vi "Teleop.vi"(10 "Match Info":T1={"Autonomous Elapsed Seconds"=0.0, "TeleOp Elapsed Seconds"=0.0, "Disabled Elapsed Seconds"=0.0, "Visited Autonomous"=FALSE, "Visited TeleOp"=FALSE, "Visited Disabled"=FALSE, "Autonomous Settings"={"Autonomous Style"=enum."Independent", "VI Refnum"=refnum}}, 11 "Call Context":T2) -> ()   [LabVIEW 2015]
doc: "This VI is called for each TeleOp packet received from the DS where the robot is not disabled. It is often used to read from the joysticks and update I/O or to update setpoints for timed control loops. It should complete and return within 20 milliseconds or it may miss DS packets."
uses:
  <vilib>/Rock Robotics/WPI/DriverStation/WPI_DriverStationDerivedRobotMode.ctl
  <vilib>/Rock Robotics/WPI/DriverStation/WPI_DriverStationMatch Info.ctl
  <vilib>/Rock Robotics/WPI/Solenoid/WPI_SolenoidValue.ctl
  <vilib>/Rock Robotics/WPI/CAN/TalonSRX/WPI_CANTalonSRX_APIControlMode.ctl
  <vilib>/Rock Robotics/WPI/Utilities/WPI_GetSetVariantRefNum.vi
  Robot Global Data.vi
  <vilib>/Rock Robotics/WPI/Solenoid/WPI_SolenoidSetEnum.vi
  <vilib>/Rock Robotics/Network Tables/NT Write Boolean.vi
  <vilib>/addons/control/pid/pid.llb/PID (DBL).vi
  <vilib>/addons/control/pid/NI_PID_pid.lvlib
panel:
  out "Shooter velocity":dbl
  out "Shooter Applied Throttle":dbl
  out "Shooter Current":dbl
  out "Arm Pot":dbl
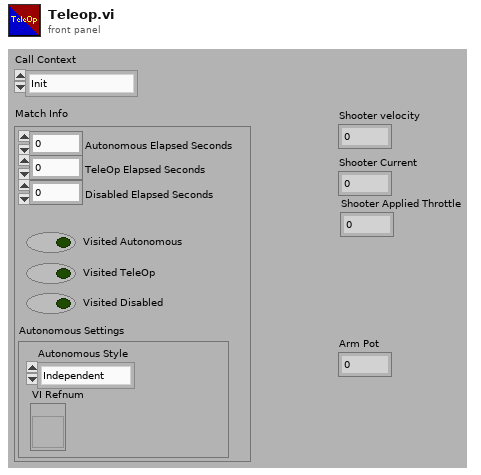
[diagram p1: front panel]
types:
  T1 = typedef "WPI_DriverStationMatch Info.ctl" = cluster{"Autonomous Elapsed Seconds":dbl, "TeleOp Elapsed Seconds":dbl, "Disabled Elapsed Seconds":dbl, "Visited Autonomous":bool, "Visited TeleOp":bool, "Visited Disabled":bool, "Autonomous Settings":cluster{"Autonomous Style":enum16{"Iterative", "Independent"}, "VI Refnum":refnum<vi>}}
  T2 = typedef "WPI_DriverStationDerivedRobotMode.ctl" = enum16{"Init", "Execute", "Stop"}
  T3 = typedef "WPI_SolenoidValue.ctl" = enum16{"Off", "On", "Forward", "Reverse"}
  T4 = typedef "WPI_JoystickDevRef.ctl" = cluster{"Device":T5}
  T5 = typedef "WPI_JoystickDeviceEnum.ctl" = enum16{"USB 0", "USB 1", "USB 2", "USB 3", "USB 4", "USB 5"}
  T6 = cluster{"Axes[0]":dbl, "Axes[1]":dbl, "Axes[2]":dbl, "Axes[3]":dbl, "Axes[4]":dbl, "Axes[5]":dbl, "Axes[6]":dbl, "Axes[7]":dbl, "Axes[8]":dbl}
  T7 = typedef "WPI_MotorControlDeviceRef.ctl" = cluster{"DeviceStatus":errorcluster, "Type":T8, "PWM":cluster{"PWM Channel":T9, "DeadBand":T10}, "CAN":cluster{"Device Number":u8, "Control Mode":T11, "Semaphore":T12, "Max Vout":dbl, "TalonSRX Control Mode":T13}, "Invert":bool}
  T8 = typedef "WPI_MotorControlType.ctl" = enum16{"PWM", "CAN", "CANTalonSRX"}
  T9 = typedef "FPGA_DIOPWMChannel.ctl" = enum8{"PWM 0", "PWM 1", "PWM 2", "PWM 3", "PWM 4", "PWM 5", "PWM 6", "PWM 7", "PWM 8", "PWM 9", "PWM MXP 0", "PWM MXP 1", "PWM MXP 2", "PWM MXP 3", "PWM MXP 4", "PWM MXP 5", "PWM MXP 6", "PWM MXP 7", "PWM MXP 8", "PWM MXP 9", "Invalid"}
  T10 = typedef "WPI_PWMDeadband.ctl" = cluster{"Name":string, "maxPositivePwm":i32, "minPositivePwm":i32, "centerPwm":i32, "maxNegativePwm":i32, "minNegativePwm":i32, "angularRange":u16}
  T11 = typedef "WPI_CANJaguar_ControlMode.ctl" = enum8{"Percent VBus", "Current", "Speed", "Position", "Voltage"}
  T12 = typedef "Semaphore RefNum" = refnum<k1>
  T13 = typedef "WPI_CANTalonSRX_APIControlMode.ctl" = enum8{"Percent VBus", "Speed", "Position", "Slave", "Unchanged / Invalid", "Voltage Compensation", "Current", "Motion Profile"}
  T14 = cluster{"Buttons[0]":bool, "Buttons[1]":bool, "Buttons[2]":bool, "Buttons[3]":bool, "Buttons[4]":bool, "Buttons[5]":bool, "Buttons[6]":bool, "Buttons[7]":bool, "Buttons[8]":bool}
  T15 = typedef "WPI_CompressorDevRef.ctl" = cluster{"DevStatus":errorcluster, "Pneumatics Control Module":u8}
  T16 = typedef "WPI_SolenoidDevRef.ctl" = cluster{"DevStatus":errorcluster, "Pneumatics Control Module":u8, "Forward Solenoid Channel":T17, "Reverse Solenoid Channel":T17}
  T17 = typedef "WPI_SolenoidChannel.ctl" = enum8{"Solenoid 0", "Solenoid 1", "Solenoid 2", "Solenoid 3", "Solenoid 4", "Solenoid 5", "Solenoid 6", "Solenoid 7", "Invalid"}
  T18 = typedef "WPI_CANTalonSRX_GlobalStatus.ctl" = cluster{"Applied Throttle":dbl, "Module Enabled":bool, "CAN Error":errorcluster, "Closed Loop Error":dbl, "Forward Limit Switch Closed":bool, "Reverse Limit Switch Closed":bool, "Sensor Position":dbl, "Sensor Velocity":dbl, "Current":dbl, "Sticky Fault - Over Temp":bool, "Sticky Fault - Under Voltage":bool, "Sticky Fault - Forward Limit":bool, "Sticky Fault - Reverse Limit":bool, "Sticky Fault - Forward Soft Limit":bool, "Sticky Fault - Reverse Soft Limit":bool, "Brake is Enabled":bool, "Encoder Position":dbl, "Encoder Velocity":dbl, "Encoder Index Count":dbl, "Encoder A Pin State":bool, "Encoder B Pin State":bool, "Encoder Index Pin State":bool, "Analog In":dbl, "Analog In Velocity":dbl, "Temperature (C)":dbl, "Battery Voltage":dbl, "Control 5 Is Supported":bool, "Current Profile Slot Select":dbl, "Pos Div 8":bool, "Vel Div 4":bool, "Pulse Width Position":i32, "Pulse Width Velocity":i32, "Pulse Width Rise To Rise (us)":i32, "Pulse Width Rise To Fall (us)":i32, "Mot Prof Active Is Under Run":bool, "Mot Prof Active Has Under Run":bool, "Mot Prof Active Is Last":bool, "Mot Prof Active Velocity Only":bool, "Mot Prof Active Is Valid":bool, "Mot Prof Buffer Is Full":bool, "Mot Prof Active Profile Slot Select":i32, "Mot Prof NextID":i32, "Mot Prof Count":i32, "Mot Prof Active Velocity":dbl, "Mot Prof Active Position":dbl, "Mot Prof Output Enable":i32}
  T19 = cluster{"proportional gain (Kc)":dbl, "integral time (Ti, min)":dbl, "derivative time (Td, min)":dbl}
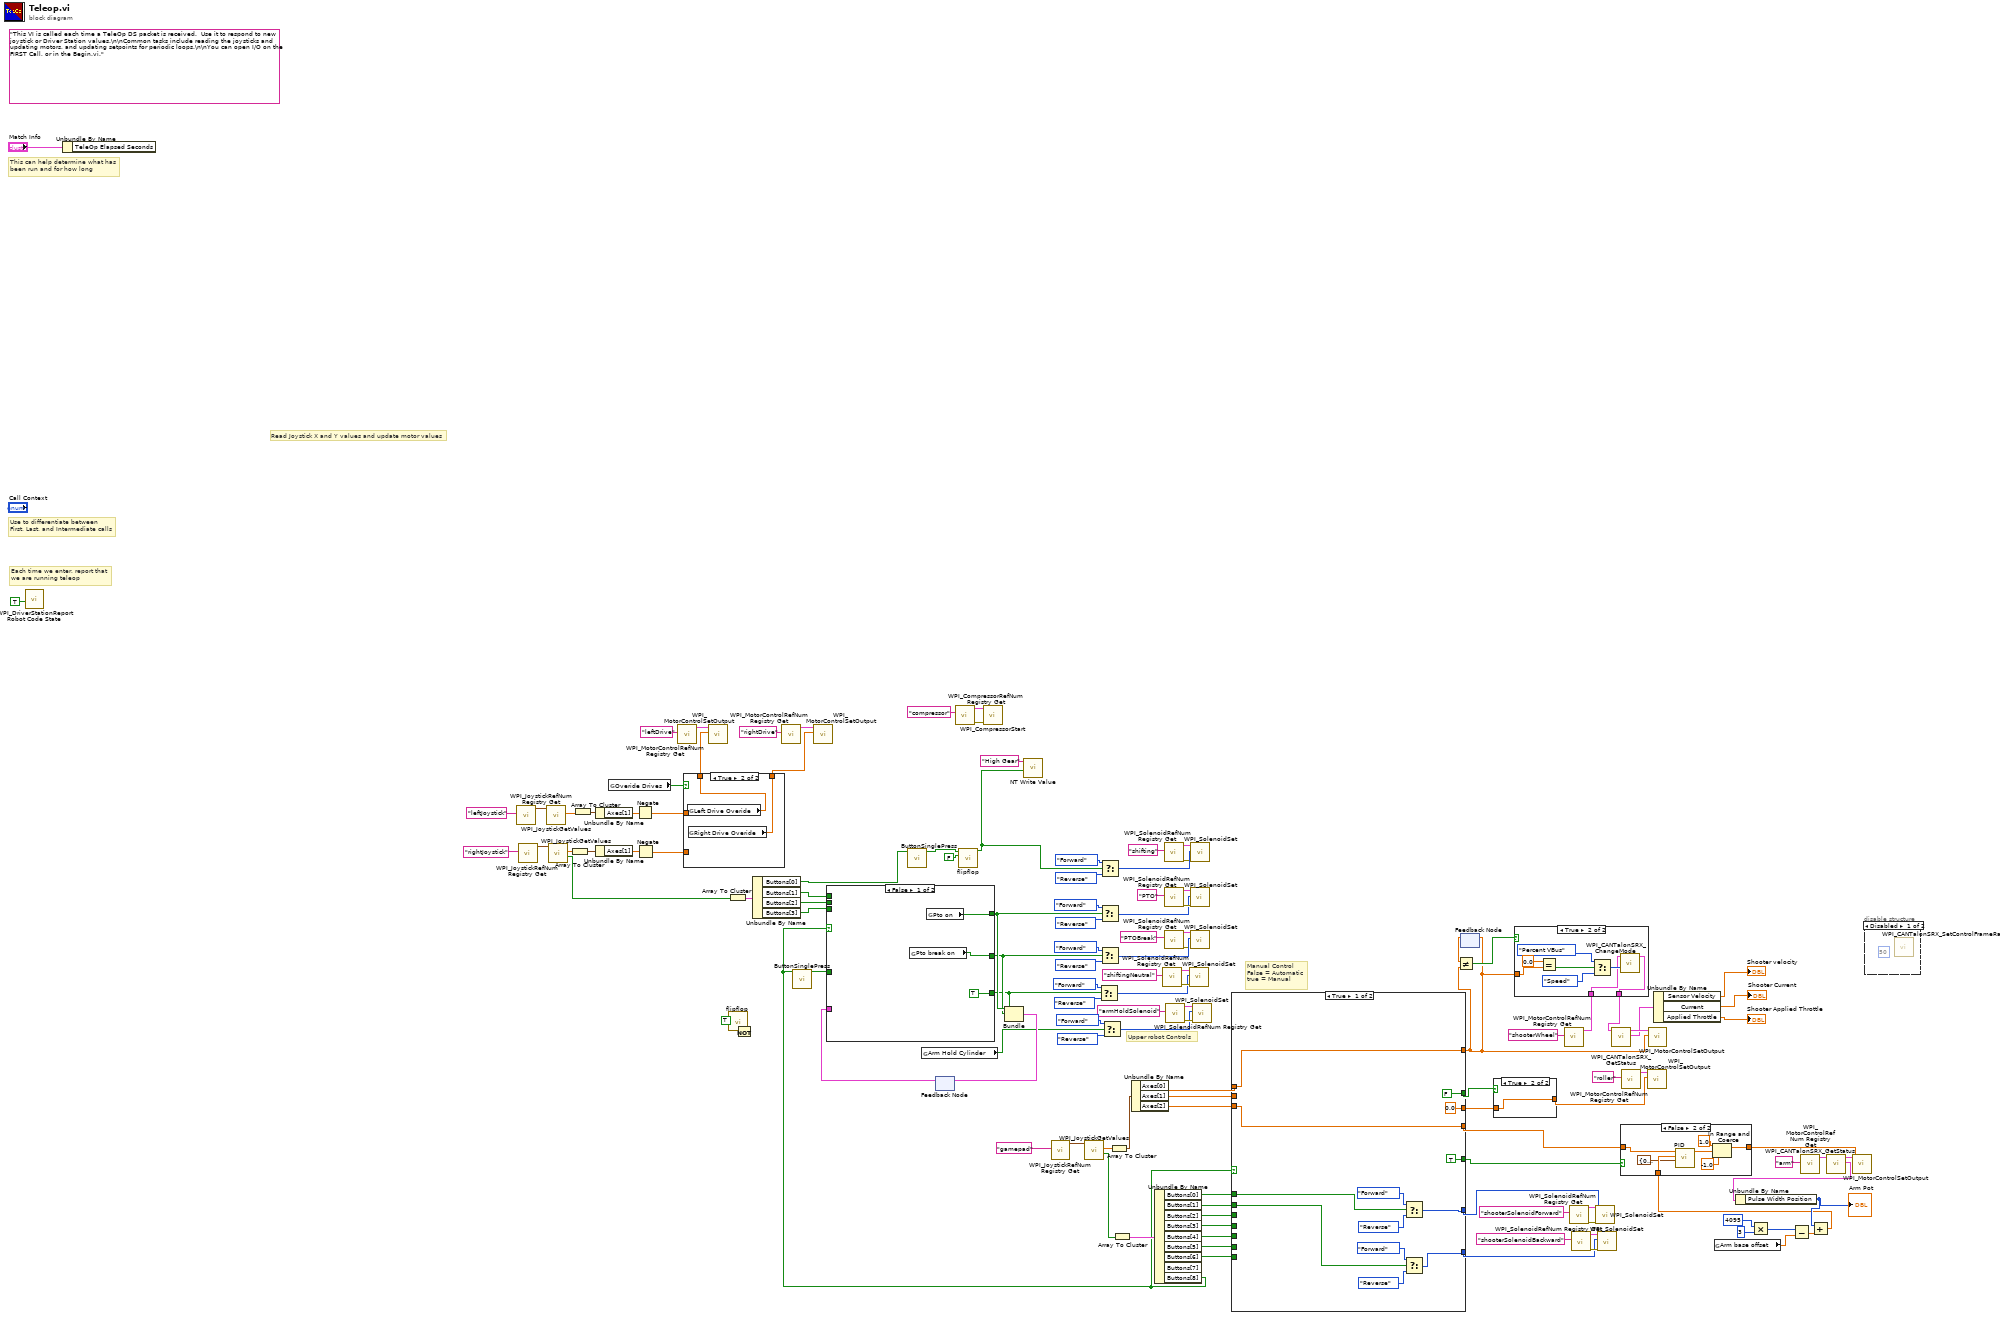
[diagram p0: block diagram]
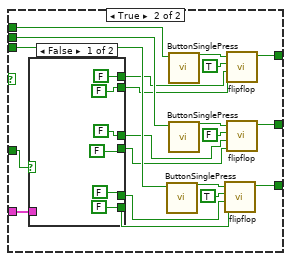
[diagram p2: hidden frame]
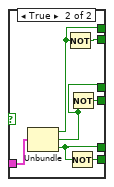
[diagram p3: hidden frame]
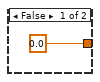
[diagram p7: hidden frame]
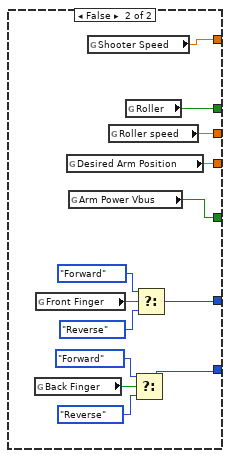
[diagram p9: hidden frame]
diagram:
  w6 = TRUE
  (unwired) "This VI is called each time a TeleOp DS packet is received.  Use it to respond to new joystick or Driver Station values.\n\nCommon tasks include reading the joysticks and updating motors, and updating setpoints for periodic loops.\n\nYou can open I/O on the FIRST Call, or in the Begin.vi."
  # "Upper robot Controls"
  # "Manual Control\nFalse = Automatic\ntrue = Manual"
  # "Read Joystick X and Y values and update motor values"
  # "Each time we enter, report that\nwe are running teleop"
  # "Use to differentiate between\nFirst, Last, and Intermediate calls"
  # "This can help determine what has\nbeen run and for how long"
  n1 = call <vilib>:"WPI_DriverStationReport Robot Code State.vi"("TeleOp"=TRUE ("Autonomous")) -> ()  [unwired: 10 in, 1 out]
  n2 = Unbundle By Name("Match Info") -> ()  [unwired: 1 out]
  n3 = call <vilib>:"WPI_JoystickRefNum Registry Get.vi"("refnum name"="leftJoystick") -> ("JoystickDevRef"=w67:T4)  [unwired: 1 in, 9 out]
  n4 = call <vilib>:"WPI_JoystickRefNum Registry Get.vi"("refnum name"="rightJoystick") -> ("JoystickDevRef"=w60:T4)  [unwired: 1 in, 9 out]
  n5 = call <vilib>:"WPI_JoystickGetValues.vi"("JoystickDevRef"=w67) -> ("Axes"=w63:dbl[])  [unwired: 6 in, 4 out]
  n6 = call <vilib>:"WPI_JoystickGetValues.vi"("JoystickDevRef"=w60) -> ("Buttons"=w58:bool[], "Axes"=w61:dbl[])  [unwired: 6 in, 3 out]
  n7 = Array To Cluster(array=w61) -> (cluster=w62:T6)
  n8 = Array To Cluster(array=w63) -> (cluster=w64:T6)
  n9 = Unbundle By Name(w64) -> ("Axes[1]"=w65:dbl)
  n10 = Unbundle By Name(w62) -> ("Axes[1]"=w57:dbl)
  n11 = global read "Robot Global Data.vi" "Overide Drives"() -> (w29:bool)
  n12 = Negate(x=w65) -> (-x=w56:dbl)
  n13 = Negate(x=w57) -> (-x=w55:dbl)
  n14 = call <vilib>:"WPI_MotorControlRefNum Registry Get.vi"("refnum name"="leftDrive") -> ("MotorControlDevRef"=w27:T7)  [unwired: 9 in, 1 out]
  n15 = case shown="True" w29 {
    tunnel: w56 -> [w130 _]
    tunnel: w55 -> [w129 _]
    tunnel: [w130 w132] -> w54
    tunnel: [w129 w131] -> w53
    frame False {
    }
    frame True {
      n16 = global read "Robot Global Data.vi" "Left Drive Overide"() -> (w132:dbl)
      n17 = global read "Robot Global Data.vi" "Right Drive Overide"() -> (w131:dbl)
    }
  }
  n18 = call <vilib>:"WPI_MotorControlSetOutput.vi"("Output"=w54, "MotorControlDevRef"=w27) -> ()  [unwired: 7 in, 3 out]
  n19 = Array To Cluster(array=w58) -> (cluster=w101:T14)
  n20 = Not(x=w6) -> (.not. x?=w7:bool)
  n21 = call "flipflop.vi"("Overide false"=w7, "Overide true"=w6) -> ()  [unwired: 9 in, 1 out]
  n22 = Unbundle By Name(w101) -> ("Buttons[0]"=w9:bool, "Buttons[1]"=w34:bool, "Buttons[2]"=w33:bool, "Buttons[3]"=w32:bool)
  n23 = call <vilib>:"WPI_MotorControlRefNum Registry Get.vi"("refnum name"="rightDrive") -> ("MotorControlDevRef"=w28:T7)  [unwired: 9 in, 1 out]
  n24 = call <vilib>:"WPI_MotorControlSetOutput.vi"("Output"=w53, "MotorControlDevRef"=w28) -> ()  [unwired: 7 in, 3 out]
  n25 = call "ButtonSinglePress.vi"("Button In"=w9) -> ("Button out"=w11:bool)  [unwired: 10 in]
  n26 = global read "Robot Global Data.vi" "Arm Hold Cylinder"() -> (w1:bool)
  n27 = feedback #1() -> (w12:cluster{"flop":bool, "flop":bool, "flop":bool})  [unwired: 1 in]
  n28 = call <vilib>:"WPI_CompressorRefNum Registry Get.vi"("refnum name"="compressor") -> ("error out"=w105:errorcluster, "CompressorDevRef"=w104:T15)  [unwired: 9 in]
  n29 = call "flipflop.vi"("Start value"=FALSE, "flip"=w11) -> ("flop"=w8:bool)  [unwired: 9 in]
  n30 = call <vilib>:"WPI_CompressorStart.vi"("error in (no error)"=w105, "CompressorDevRef"=w104) -> ()  [unwired: 8 in, 2 out]
  n31 = call-poly <vilib>:"NT Write Value.vi"("Boolean"=w8, "Name"="High Gear") -> ()  [unwired: 9 in, 1 out]
  n32 = call <vilib>:"WPI_JoystickRefNum Registry Get.vi"("refnum name"="gamepad") -> ("JoystickDevRef"=w122:T4)  [unwired: 1 in, 9 out]
  n33 = call <vilib>:"WPI_JoystickGetValues.vi"("JoystickDevRef"=w122) -> ("Buttons"=w123:bool[], "Axes"=w112:dbl[])  [unwired: 6 in, 3 out]
  n34 = Select(t=WPI_SolenoidValue."Forward" ("Value"), s=w8, f=WPI_SolenoidValue."Reverse" ("Value")) -> (s? t:f=w80:T3)
  n35 = Select(t=WPI_SolenoidValue."Forward" ("Value"), s=w1, f=WPI_SolenoidValue."Reverse" ("Value")) -> (s? t:f=w17:T3)
  n36 = Array To Cluster(array=w112) -> (cluster=w111:T6)
  n37 = Array To Cluster(array=w123) -> (cluster=w124:T14)
  n38 = Unbundle By Name(w111) -> ("Axes[0]"=w110:dbl, "Axes[1]"=w109:dbl, "Axes[2]"=w108:dbl)
  n39 = Unbundle By Name(w124) -> ("Buttons[0]"=w107:bool, "Buttons[1]"=w106:bool, "Buttons[2]"=w117:bool, "Buttons[3]"=w116:bool, "Buttons[4]"=w115:bool, "Buttons[5]"=w114:bool, "Buttons[6]"=w113:bool, "Buttons[8]"=w5:bool)  [unwired: 1 out]
  n40 = call "ButtonSinglePress.vi"("Button In"=w5) -> ("Button out"=w4:bool)  [unwired: 10 in]
  n41 = case shown="False" w5 {
    tunnel: [w135 w155] -> w16
    tunnel: [w134 w150] -> w15
    tunnel: [TRUE w149] -> w14
    tunnel: w34 -> [_ w146]
    tunnel: w33 -> [_ w145]
    tunnel: w32 -> [_ w144]
    tunnel: w12 -> [_ w142]
    tunnel: w4 -> [_ w143]
    frame False {
      n42 = global read "Robot Global Data.vi" "Pto break on"() -> (w134:bool)
      n43 = global read "Robot Global Data.vi" "Pto on"() -> (w135:bool)
    }
    frame True {
      n44 = case shown="False" w143 {
        tunnel: w142 -> [_ w168]
        tunnel: [FALSE ("flop") w167] -> w140
        tunnel: [FALSE ("flop") w166] -> w141
        tunnel: [FALSE ("flop") w165] -> w138
        tunnel: [FALSE ("flop") w164] -> w139
        tunnel: [FALSE ("flop") w163] -> w137
        tunnel: [FALSE ("flop") w162] -> w136
        frame False {
        }
        frame True {
          n45 = Unbundle(w168) -> ("flop"=w166:bool, "flop"=w165:bool, "flop"=w163:bool)
          n46 = Not(x=w166) -> (.not. x?=w167:bool)
          n47 = Not(x=w163) -> (.not. x?=w162:bool)
          n48 = Not(x=w165) -> (.not. x?=w164:bool)
        }
      }
      n49 = call "ButtonSinglePress.vi"("Button In"=w144) -> ("Button out"=w148:bool)  [unwired: 10 in]
      n50 = call "ButtonSinglePress.vi"("Button In"=w146) -> ("Button out"=w154:bool)  [unwired: 10 in]
      n51 = call "ButtonSinglePress.vi"("Button In"=w145) -> ("Button out"=w151:bool)  [unwired: 10 in]
      n52 = call "flipflop.vi"("Overide false"=w136, "Overide true"=w137, "Start value"=TRUE, "flip"=w148) -> ("flop"=w149:bool)  [unwired: 7 in]
      n53 = call "flipflop.vi"("Overide false"=w140, "Overide true"=w141, "Start value"=TRUE, "flip"=w154) -> ("flop"=w155:bool)  [unwired: 7 in]
      n54 = call "flipflop.vi"("Overide false"=w139, "Overide true"=w138, "Start value"=FALSE, "flip"=w151) -> ("flop"=w150:bool)  [unwired: 7 in]
    }
  }
  n55 = Bundle("flop"=w16, "flop"=w15, "flop"=w14) -> (w13:cluster{"flop":bool, "flop":bool, "flop":bool})  [unwired: 1 in]
  n56 = feedback-in #1(w13) -> ()
  n57 = Select(t=WPI_SolenoidValue."Forward" ("Value"), s=w14, f=WPI_SolenoidValue."Reverse" ("Value")) -> (s? t:f=w37:T3)
  n58 = Select(t=WPI_SolenoidValue."Forward" ("Value"), s=w16, f=WPI_SolenoidValue."Reverse" ("Value")) -> (s? t:f=w49:T3)
  n59 = Select(t=WPI_SolenoidValue."Forward" ("Value"), s=w15, f=WPI_SolenoidValue."Reverse" ("Value")) -> (s? t:f=w44:T3)
  n60 = call <vilib>:"WPI_SolenoidRefNum Registry Get.vi"("refnum name"="shiftingNeutral") -> ("error out"=w40:errorcluster, "SolenoidDevRef"=w39:T16)  [unwired: 9 in]
  n61 = call <vilib>:"WPI_SolenoidRefNum Registry Get.vi"("refnum name"="PTO") -> ("error out"=w52:errorcluster, "SolenoidDevRef"=w51:T16)  [unwired: 9 in]
  n62 = call <vilib>:"WPI_SolenoidRefNum Registry Get.vi"("refnum name"="PTOBreak") -> ("error out"=w41:errorcluster, "SolenoidDevRef"=w42:T16)  [unwired: 9 in]
  n63 = call <vilib>:"WPI_SolenoidRefNum Registry Get.vi"("refnum name"="shifting") -> ("error out"=w77:errorcluster, "SolenoidDevRef"=w78:T16)  [unwired: 9 in]
  n64 = call <vilib>:"WPI_SolenoidRefNum Registry Get.vi"("refnum name"="armHoldSolenoid") -> ("error out"=w18:errorcluster, "SolenoidDevRef"=w2:T16)  [unwired: 9 in]
  n65 = call-poly <vilib>:"WPI_SolenoidSet.vi"("error in (no error)"=w40, "Value"=w37, "SolenoidDevRef"=w39) -> ()  [unwired: 7 in, 2 out]
  n66 = call-poly <vilib>:"WPI_SolenoidSet.vi"("error in (no error)"=w52, "Value"=w49, "SolenoidDevRef"=w51) -> ()  [unwired: 7 in, 2 out]
  n67 = call-poly <vilib>:"WPI_SolenoidSet.vi"("error in (no error)"=w41, "Value"=w44, "SolenoidDevRef"=w42) -> ()  [unwired: 7 in, 2 out]
  n68 = call-poly <vilib>:"WPI_SolenoidSet.vi"("error in (no error)"=w77, "Value"=w80, "SolenoidDevRef"=w78) -> ()  [unwired: 7 in, 2 out]
  n69 = call-poly <vilib>:"WPI_SolenoidSet.vi"("error in (no error)"=w18, "Value"=w17, "SolenoidDevRef"=w2) -> ()  [unwired: 7 in, 2 out]
  n70 = case shown="True" w5 {
    tunnel: w117 -> [_ _]
    tunnel: w116 -> [_ _]
    tunnel: w115 -> [_ _]
    tunnel: w114 -> [_ _]
    tunnel: w113 -> [_ _]
    tunnel: w110 -> [w175 _]
    tunnel: w109 -> [_ _]
    tunnel: w108 -> [w174 _]
    tunnel: [w174 w184] -> w84
    tunnel: [w175 w186] -> w22
    tunnel: [w178 w188] -> w76
    tunnel: [w177 w187] -> w83
    tunnel: w107 -> [w173 _]
    tunnel: w106 -> [w172 _]
    tunnel: [FALSE w185] -> w68
    tunnel: [TRUE ("Arm Power Vbus") w183] -> w74
    tunnel: [0.0 ("Roller speed") w182] -> w31
    frame True {
      n71 = Select(t=WPI_SolenoidValue."Forward" ("Value"), s=w173, f=WPI_SolenoidValue."Reverse" ("Value")) -> (s? t:f=w178:T3)
      n72 = Select(t=WPI_SolenoidValue."Forward" ("Value"), s=w172, f=WPI_SolenoidValue."Reverse" ("Value")) -> (s? t:f=w177:T3)
    }
    frame False {
      n73 = global read "Robot Global Data.vi" "Back Finger"() -> (w191:bool)
      n74 = global read "Robot Global Data.vi" "Front Finger"() -> (w192:bool)
      n75 = global read "Robot Global Data.vi" "Desired Arm Position"() -> (w184:dbl)
      n76 = global read "Robot Global Data.vi" "Arm Power Vbus"() -> (w183:bool)
      n77 = global read "Robot Global Data.vi" "Shooter Speed"() -> (w186:dbl)
      n78 = global read "Robot Global Data.vi" "Roller speed"() -> (w182:dbl)
      n79 = global read "Robot Global Data.vi" "Roller"() -> (w185:bool)
      n80 = Select(t=WPI_SolenoidValue."Forward" ("Value"), s=w191, f=WPI_SolenoidValue."Reverse" ("Value")) -> (s? t:f=w187:T3)
      n81 = Select(t=WPI_SolenoidValue."Forward" ("Value"), s=w192, f=WPI_SolenoidValue."Reverse" ("Value")) -> (s? t:f=w188:T3)
    }
  }
  n82 = feedback-in #2(w22) -> ()
  n83 = feedback #2() -> (w24:dbl)  [unwired: 1 in]
  n84 = Not Equal?(x=w24, y=w22) -> (x != y?=w23:bool)
  n85 = case shown="True" w68 {
    tunnel: [0.0 w196] -> w30
    tunnel: w31 -> [_ w196]
    frame False {
    }
    frame True {
    }
  }
  n86 = call <vilib>:"WPI_MotorControlRefNum Registry Get.vi"("refnum name"="shooterWheel") -> ("MotorControlDevRef"=w26:T7)  [unwired: 9 in, 1 out]
  n87 = case shown="True" w23 {
    tunnel: w26 -> [w197 w202]
    tunnel: [w197 w201] -> w25
    tunnel: w22 -> [_ w200]
    frame False {
    }
    frame True {
      n88 = Equal?(x=0.0, y=w200) -> (x = y?=w199:bool)
      n89 = Select(t=WPI_CANTalonSRX_APIControlMode."Percent VBus" ("Control Mode"), s=w199, f=WPI_CANTalonSRX_APIControlMode."Speed" ("Control Mode")) -> (s? t:f=w203:T13)
      n90 = call <vilib>:"WPI_CANTalonSRX_ChangeMode.vi"("Control Mode"=w203, "CAN Talon SRX Ref"=w202) -> ("CAN Talon SRX Ref"=w201:T7)  [unwired: 8 in, 1 out]
    }
  }
  n91 = call <vilib>:"WPI_SolenoidRefNum Registry Get.vi"("refnum name"="shooterSolenoidForward") -> ("error out"=w95:errorcluster, "SolenoidDevRef"=w96:T16)  [unwired: 9 in]
  n92 = call <vilib>:"WPI_SolenoidRefNum Registry Get.vi"("refnum name"="shooterSolenoidBackward") -> ("error out"=w98:errorcluster, "SolenoidDevRef"=w99:T16)  [unwired: 9 in]
  n93 = call-poly <vilib>:"WPI_SolenoidSet.vi"("error in (no error)"=w95, "Value"=w76, "SolenoidDevRef"=w96) -> ()  [unwired: 7 in, 2 out]
  n94 = call-poly <vilib>:"WPI_SolenoidSet.vi"("error in (no error)"=w98, "Value"=w83, "SolenoidDevRef"=w99) -> ()  [unwired: 7 in, 2 out]
  n95 = call <vilib>:"WPI_CANTalonSRX_GetStatus.vi"("CAN Talon SRX Ref"=w25) -> ("Talon SRX Status"=w72:T18, "CAN Talon SRX Ref"=w73:T7)  [unwired: 8 in, 1 out]
  n96 = call <vilib>:"WPI_MotorControlRefNum Registry Get.vi"("refnum name"="roller") -> ("MotorControlDevRef"=w118:T7)  [unwired: 9 in, 1 out]
  n97 = call <vilib>:"WPI_MotorControlSetOutput.vi"("Output"=w30, "MotorControlDevRef"=w118) -> ()  [unwired: 7 in, 3 out]
  n98 = call <vilib>:"WPI_MotorControlSetOutput.vi"("Output"=w22, "MotorControlDevRef"=w73) -> ()  [unwired: 7 in, 3 out]
  n99 = Unbundle By Name(w72) -> ("Sensor Velocity"=→"Shooter velocity":dbl, "Current"=→"Shooter Current":dbl, "Applied Throttle"=→"Shooter Applied Throttle":dbl)
  n100 = global read "Robot Global Data.vi" "Arm base offset"() -> (w88:dbl)
  n101 = Multiply(x=4095, y=3) -> (x*y=w89:i32)
  n102 = Subtract(x=w89, y=w88) -> (x-y=w87:dbl)
  n103 = call <vilib>:"WPI_MotorControlRefNum Registry Get.vi"("refnum name"="arm") -> ("MotorControlDevRef"=w94:T7)  [unwired: 9 in, 1 out]
  n104 = call <vilib>:"WPI_CANTalonSRX_GetStatus.vi"("CAN Talon SRX Ref"=w94) -> ("Talon SRX Status"=w93:T18, "CAN Talon SRX Ref"=w75:T7)  [unwired: 8 in, 1 out]
  n105 = Unbundle By Name(w93) -> ("Pulse Width Position"=w86:i32)
  "Arm Pot" <- w86
  n106 = Add(x=w86, y=w87) -> (x+y=w85:dbl)
  n107 = case shown="False" w74 {
    tunnel: [w206 w210] -> w92
    tunnel: w85 -> [_ w209]
    tunnel: w84 -> [w206 w208]
    frame True {
    }
    frame False {
      n108 = call-poly <vilib>:"PID.vi"("PID gains"=T19 {"proportional gain (Kc)"=0.0005, "integral time (Ti, min)"=0.0, "derivative time (Td, min)"=0.0}, "process variable"=w209, "setpoint"=w208) -> ("output"=w213:dbl)  [unwired: 7 in, 1 out]
      n109 = In Range and Coerce(upper limit=1.0, x=w213, lower limit=-1.0) -> (coerced(x)=w210:dbl)  [unwired: 1 out]
    }
  }
  n110 = call <vilib>:"WPI_MotorControlSetOutput.vi"("Output"=w92, "MotorControlDevRef"=w75) -> ()  [unwired: 7 in, 3 out]
  n111 = disable-structure shown="Disabled" {
    frame Disabled {
      (unwired) u8 50 ("Control Frame Rate (ms)")
      n112 = call <vilib>:"WPI_CANTalonSRX_SetControlFrameRate.vi"() -> ()  [unwired: 10 in, 2 out]
    }
    frame Enabled {
    }
  }
